vi "E06_FiltroEMA.vi"() -> ()   [LabVIEW 2026]
uses:
  <vilib>/Analysis/NI_AALBase.lvlib
panel:
  out "Waveform Chart":dbl(graph)
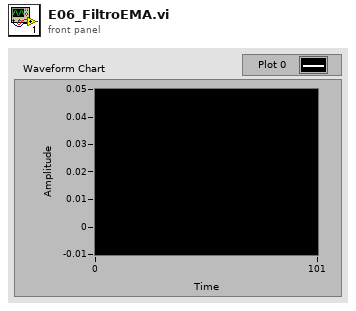
[diagram p1: front panel]
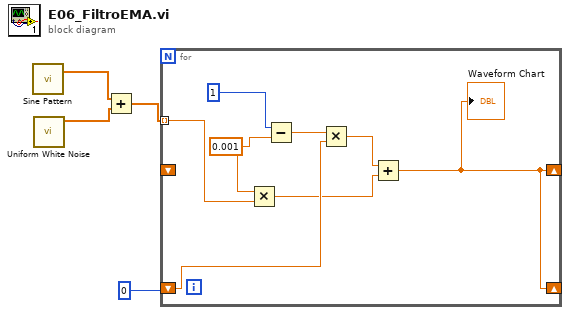
[diagram p0: block diagram]
diagram:
  n1 = call <vilib>:"Sine Pattern.vi"() -> ("Sinusoidal Pattern"=w3:dbl[])  [unwired: 4 in, 1 out]
  n2 = call <vilib>:"Uniform White Noise.vi"() -> ("uniform white noise"=w4:dbl[])  [unwired: 10 in, 1 out]
  n3 = Add(x=w3, y=w4) -> (x+y=w2:dbl[])
  n4 = for {
    tunnel: w2 -> [w10] mode=indexing
    shift-right: [w5] -> _
    shift-left: 0 -> [w8]
    shift-right: [w5] -> _
    shift-left: _ -> [_]
    w11 = 0.001
    n5 = Multiply(x=w11, y=w10) -> (x*y=w7:dbl)
    n6 = Subtract(x=1, y=w11) -> (x-y=w9:dbl)
    n7 = Multiply(x=w9, y=w8) -> (x*y=w6:dbl)
    n8 = Add(x=w6, y=w7) -> (x+y=w5:dbl)
    "Waveform Chart" <- w5
  }
